vi "Read Server Internal UEs.vi"(8 "error in (no error)":errorcluster, 11 "SignalGeneratorService in":refnum<class "I2C.lvclass">) -> (0 "error out":errorcluster, 2 "Server Internal UEs":T1, 3 "SignalGeneratorService out":refnum<class "I2C.lvclass">)   [LabVIEW 2021, in "Unary_server.lvlib" / "I2C.lvclass"]
uses:
  I2C.lvclass
  typeDefs/Server Internal UEs.ctl
  typeDefs/Server Internal Message.ctl
  I2C.lvclass/I2C.ctl
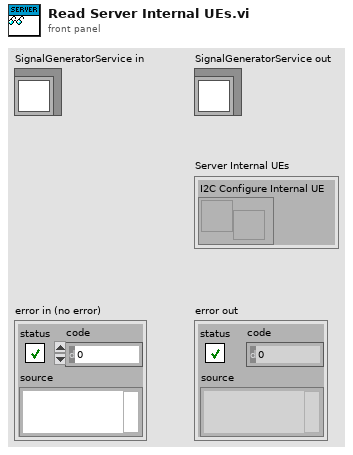
[diagram p1: front panel]
types:
  T1 = typedef "Unary_server.lvlib/I2C.lvclass/Server Internal UEs.ctl" = cluster{"I2C Configure Internal UE":refnum<user-event>}
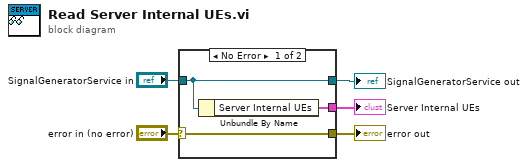
[diagram p0: block diagram]
diagram:
  n1 = case shown="No Error" "error in (no error)" {
    selector: "error in (no error)" -> [w8 w9]
    tunnel: [w8 w9] -> w4
    tunnel: [w7 w10] -> w2
    tunnel: "SignalGeneratorService in" -> [w7 w10]
    tunnel: [w6 _] -> w1
    frame No Error {
      n2 = Unbundle By Name(w7) -> ("Server Internal UEs"=w6:T1)
    }
    frame Error {
    }
  }
  "error out" <- w4
  "SignalGeneratorService out" <- w2
  "Server Internal UEs" <- w1
